vi "get device interface info.vi"(8 "error in (no error)":errorcluster, 10 "Device Info in":T1={"Interface Data"={"Name"="", "Unit ID"=0, "Refresh Rate"=0, "Write Rate"=0, "Write Mode"=enum."Value Change", "Interface Type"=enum."TCP Master", "TCP Settings"={"Address"="", "Port"=0, "Timeout"=0}, "Serial Settings"={"VISA resource name"="", "baud rate"=0, "parity (even)"=0, "flow control (none)"=0, "serial type"=enum."RTU", "Wire Mode"=-1}}, "Modbus Input Groups"=[], "Modbus Output Groups"=[], "error in (no error)"={"status"=FALSE, "code"=0, "source"=""}, "Modbus Input Engine Group Names"=[], "Modbus Output Engine Group Names"=[]} {"Interface Data"."Serial Settings"."Wire Mode" items=["Unknown"=-1, "RS485/Wire4"=0, "RS485/Wire2-EchoDTR"=1, "RS485/Wire2-CtrlDTR"=2, "RS485/Wire2-Auto"=3, "RS232/DTE"=128, "RS232/DCE"=129, "RS232/AUTO"=130]; "Interface Data"."Serial Settings"."parity (even)" items=["None", "Odd", "Even", "Mark", "Space"]; "Interface Data"."Serial Settings"."flow control (none)" items=["None", "XON/XOFF", "RTS/CTS", "XON/XOFF & RTS/CTS", "DTR/DSR", "XON/XOFF & DTR/DSR"]}, 11 "Device Item Ref in in":T12 format="%.0x") -> (0 "error out":errorcluster, 2 "Device Info out":T1={"Interface Data"={"Name"="", "Unit ID"=0, "Refresh Rate"=0, "Write Rate"=0, "Write Mode"=enum."Value Change", "Interface Type"=enum."TCP Master", "TCP Settings"={"Address"="", "Port"=0, "Timeout"=0}, "Serial Settings"={"VISA resource name"="", "baud rate"=0, "parity (even)"=0, "flow control (none)"=0, "serial type"=enum."RTU", "Wire Mode"=-1}}, "Modbus Input Groups"=[], "Modbus Output Groups"=[], "error in (no error)"={"status"=FALSE, "code"=0, "source"=""}, "Modbus Input Engine Group Names"=[], "Modbus Output Engine Group Names"=[]} {"Interface Data"."Serial Settings"."Wire Mode" items=["Unknown"=-1, "RS485/Wire4"=0, "RS485/Wire2-EchoDTR"=1, "RS485/Wire2-CtrlDTR"=2, "RS485/Wire2-Auto"=3, "RS232/DTE"=128, "RS232/DCE"=129, "RS232/AUTO"=130]; "Interface Data"."Serial Settings"."parity (even)" items=["None", "Odd", "Even", "Mark", "Space"]; "Interface Data"."Serial Settings"."flow control (none)" items=["None", "XON/XOFF", "RTS/CTS", "XON/XOFF & RTS/CTS", "DTR/DSR", "XON/XOFF & DTR/DSR"]}, 3 "Device Item Ref out":T12 format="%.0x")   [LabVIEW 2015, in "Modbus Master System Explorer.lvlib"]
uses:
  Modbus Master System Explorer.lvlib
  <vilib>/NI Veristand/Custom Device API/Custom Device Item Ref.ctl
  Shared/Device Info.ctl
  Shared/Write Mode.ctl
  Shared/Controls/Interface Type.ctl
  Shared/Controls/Data Model/TCP Settings.ctl
  Shared/Controls/Data Model/Serial Settings.ctl
  Engine/SubVIs/Bulk Data Access.ctl
  Modbus Type.ctl
  Shared/Controls/Data Model/Channel.ctl
  <vilib>/NI Veristand/Custom Device API/Custom Device Channel Type.ctl
  Shared/Controls/Data Model/Mapping.ctl
  Shared/Controls/Data Model/DataType.ctl
  Shared/Modbus Master Shared.lvlib
  <vilib>/NI VeriStand/Custom Device API/Custom Device API.lvlib
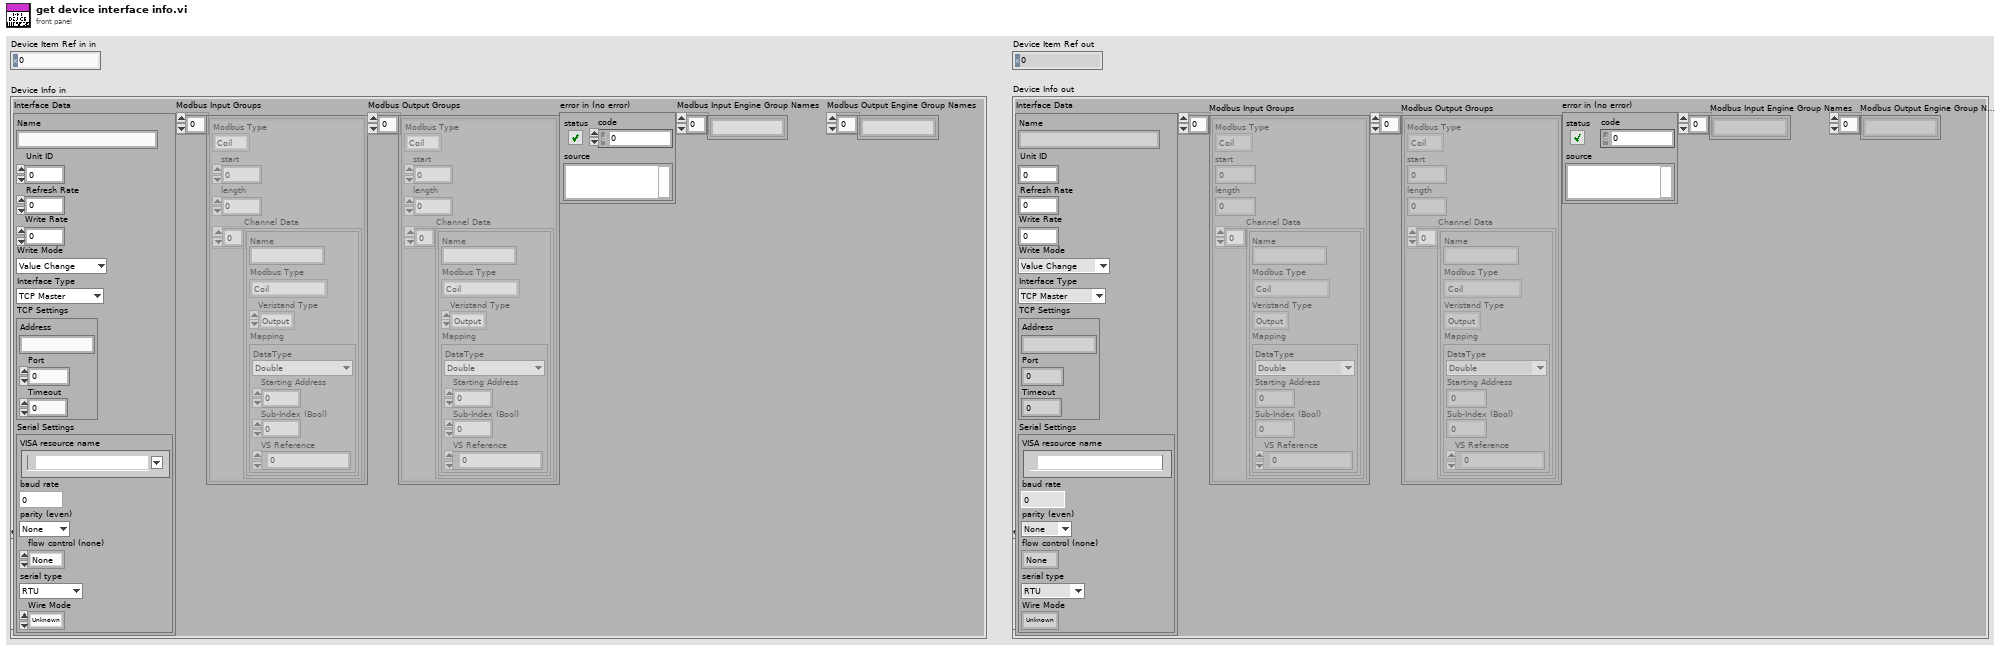
[diagram p1: front panel]
types:
  T1 = typedef "Modbus Master Shared.lvlib/Device Info.ctl" = cluster{"Interface Data":cluster{"Name":string, "Unit ID":u8, "Refresh Rate":i32, "Write Rate":i32, "Write Mode":T2, "Interface Type":T3, "TCP Settings":T4, "Serial Settings":T5}, "Modbus Input Groups":T6[], "Modbus Output Groups":T6[], "error in (no error)":errorcluster, "Modbus Input Engine Group Names":string[], "Modbus Output Engine Group Names":string[]}
  T2 = typedef "Modbus Master Shared.lvlib/Write Mode.ctl" = enum16{"Value Change", "Interval"}
  T3 = typedef "Modbus Master Shared.lvlib/Interface Type.ctl" = enum16{"TCP Master", "Serial Master", "TCP Slave", "Serial Slave"}
  T4 = typedef "Modbus Master Shared.lvlib/TCP Settings.ctl" = cluster{"Address":string, "Port":u16, "Timeout":i32}
  T5 = typedef "Modbus Master Shared.lvlib/Serial Settings.ctl" = cluster{"VISA resource name":refnum<visa-resource-name>, "baud rate":u32, "parity (even)":u16, "flow control (none)":u16, "serial type":enum16{"RTU", "ASCII"}, "Wire Mode":i16}
  T6 = typedef "Modbus Master Shared.lvlib/Bulk Data Access.ctl" = cluster{"Modbus Type":T7, "start":u16, "length":u16, "Channel Data":T8[]}
  T7 = typedef "Modbus Master Shared.lvlib/Modbus Type.ctl" = enum16{"Coil", "Discrete Input", "Holding Register", "Input Register"}
  T8 = typedef "Modbus Master Shared.lvlib/Channel.ctl" = cluster{"Name":string, "Modbus Type":T7, "Veristand Type":T9, "Mapping":T10}
  T9 = typedef "Custom Device API.lvlib/Custom Device Channel Type.ctl" = enum16{"Input", "Output"}
  T10 = typedef "Modbus Master Shared.lvlib/Mapping.ctl" = cluster{"DataType":T11, "Starting Address":u16, "Sub-Index (Bool)":u16, "VS Reference":T12}
  T11 = typedef "Modbus Master Shared.lvlib/DataType.ctl" = enum16{"Double", "Single", "I64", "I32", "I16", "I8", "U64", "U32", "U16", "U8", "Boolean"}
  T12 = typedef "Custom Device API.lvlib/Custom Device Item Ref.ctl" = u64
  T13 = typedef "Modbus Master Shared.lvlib/Parity.ctl" = u16
  T14 = typedef "Modbus Master Shared.lvlib/Serial Type.ctl" = enum16{"RTU", "ASCII"}
  T15 = typedef "Modbus Master Shared.lvlib/Flow Control.ctl" = u16
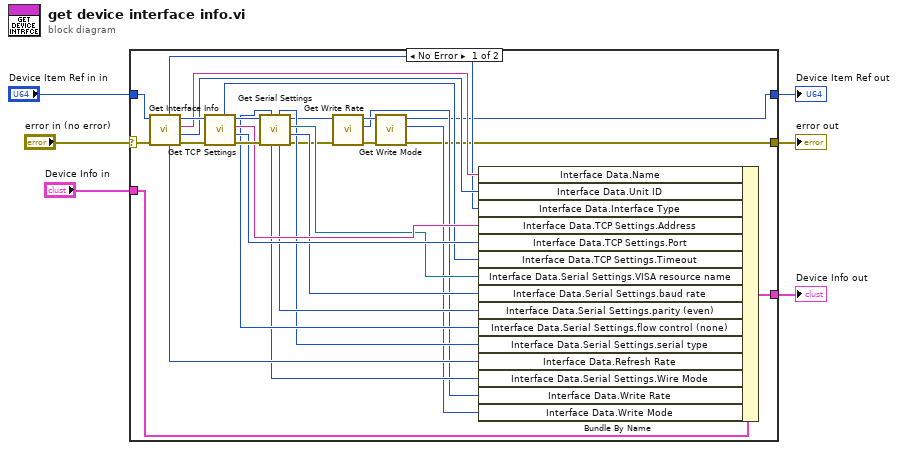
[diagram p0: block diagram]
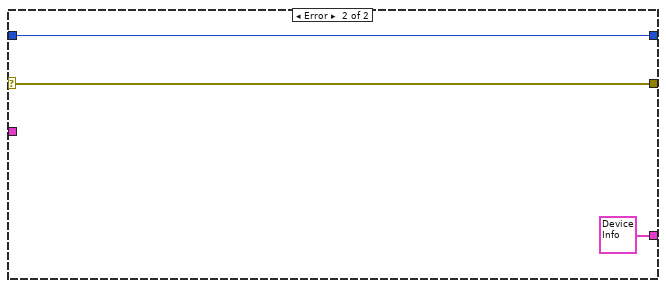
[diagram p2: hidden frame]
diagram:
  n1 = case shown="No Error" "error in (no error)" {
    selector: "error in (no error)" -> [w18 w37]
    tunnel: [w31 T1 {"Interface Data"={"Name"="", "Unit ID"=0, "Refresh Rate"=0, "Write Rate"=0, "Write Mode"=enum."Value Change", "Interface Type"=enum."TCP Master", "TCP Settings"={"Address"="", "Port"=0, "Timeout"=0}, "Serial Settings"={"VISA resource name"="", "baud rate"=9600, "parity (even)"=2, "flow control (none)"=0, "serial type"=enum."RTU", "Wire Mode"=-1}}, "Modbus Input Groups"=[], "Modbus Output Groups"=[], "error in (no error)"={"status"=FALSE, "code"=0, "source"=""}, "Modbus Input Engine Group Names"=[], "Modbus Output Engine Group Names"=[]} ("Device Info in")] -> w2
    tunnel: "Device Item Ref in in" -> [w20 w38]
    tunnel: [w9 w38] -> w4
    tunnel: [w7 w37] -> w6
    tunnel: "Device Info in" -> [w17 _]
    frame No Error {
      n2 = call "Get Interface Info.vi"("error in (no error)"=w18, "Device Item Ref in"=w20) -> ("error out"=w33:errorcluster, "Unit ID"=w29:u16, "Name"=w30:string, "Item Ref out"=w32:T12, "Refresh Rate"=w19:i32, "Interface Type"=w28:T3)  [unwired: 4 in]
      n3 = call "Get TCP Settings.vi"("error in (no error)"=w33, "Item Ref in"=w32) -> ("error out"=w35:errorcluster, "Port"=w26:u16, "Address"=w27:string, "Item Ref out"=w34:T12, "Timeout"=w16:i32)  [unwired: 5 in]
      n4 = call "Get Serial Settings.vi"("error in (no error)"=w35, "Item Ref in"=w34) -> ("error out"=w8:errorcluster, "baud rate"=w24:u32, "VISA resource name"=w25:refnum<visa-resource-name>, "Item Ref out"=w10:T12, "parity (even)"=w23:T13, "serial type"=w21:T14, "Wire Mode"=w15:i32, "flow control (none)"=w22:T15)  [unwired: 2 in]
      n5 = call "Get Write Rate.vi"("error in (no error)"=w8, "Item Ref in"=w10) -> ("error out"=w13:errorcluster, "Value"=w12:i32, "Item Ref out"=w14:T12)  [unwired: 7 in]
      n6 = call "Get Write Mode.vi"("error in (no error)"=w13, "Item Ref in"=w14) -> ("error out"=w7:errorcluster, "Write Mode"=w11:T2, "Item Ref out"=w9:T12)  [unwired: 7 in]
      n7 = Bundle By Name(cluster=w17, "Interface Data.Name"=w30, "Interface Data.Unit ID"=w29, "Interface Data.Interface Type"=w28, "Interface Data.TCP Settings.Address"=w27, "Interface Data.TCP Settings.Port"=w26, "Interface Data.TCP Settings.Timeout"=w16, "Interface Data.Serial Settings.VISA resource name"=w25, "Interface Data.Serial Settings.baud rate"=w24, "Interface Data.Serial Settings.parity (even)"=w23, "Interface Data.Serial Settings.flow control (none)"=w22, "Interface Data.Serial Settings.serial type"=w21, "Interface Data.Refresh Rate"=w19, "Interface Data.Serial Settings.Wire Mode"=w15, "Interface Data.Write Rate"=w12, "Interface Data.Write Mode"=w11) -> (w31:T1)
    }
    frame Error {
    }
  }
  "error out" <- w6
  "Device Item Ref out" <- w4
  "Device Info out" <- w2
